vi "IMAQdx Reset Camera.vi"(7 "Reset All? (No)":bool, 8 "error in":errorcluster, 11 "Session In":T1) -> (0 "error out":errorcluster)   [LabVIEW 2020, in "NI_Vision_Acquisition_Software.lvlib"]
doc: "Performs a manual reset on a camera. Stops any ongoing acquisitions."
uses:
  NI_Vision_Acquisition_Software.lvlib
  IMAQdx.ctl
  niimaqdx.dll
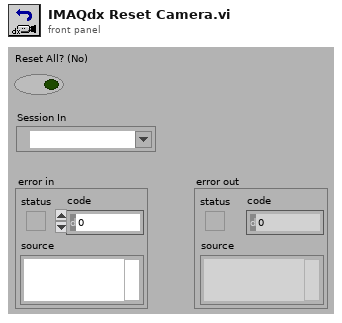
[diagram p1: front panel]
types:
  T1 = typedef "IMAQdx.ctl" = refnum<k21>
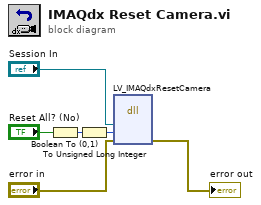
[diagram p0: block diagram]
diagram:
  n1 = Boolean To (0,1)(Boolean="Reset All? (No)") -> (0, 1=w5:i16)
  n2 = To Unsigned Long Integer(number=w5) -> (unsigned 32bit integer=w4:u32)
  n3 = dll-call lib="niimaqdx.dll" fn="LV_IMAQdxResetCamera"("interfaceName"="Session In", "resetAll"=w4, "error in"="error in") -> ("error in"=→"error out":errorcluster)  [unwired: 6 in, 2 out]
